vi "X_2.91_main.vi"() -> ()   [LabVIEW 2022 SP3]
panel:
  in  "stop":bool
  in  "Login":bool
  out "Status":string
  out "usr_db":string
  in  "usr":string
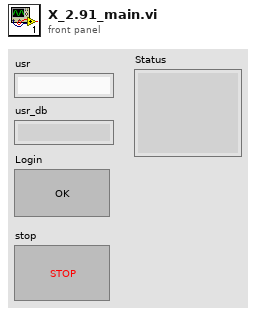
[diagram p1: front panel]
types:
  T1 = enum32{"Invalid", "Standard", "Closed", "Hidden", "Minimized", "Maximized"}
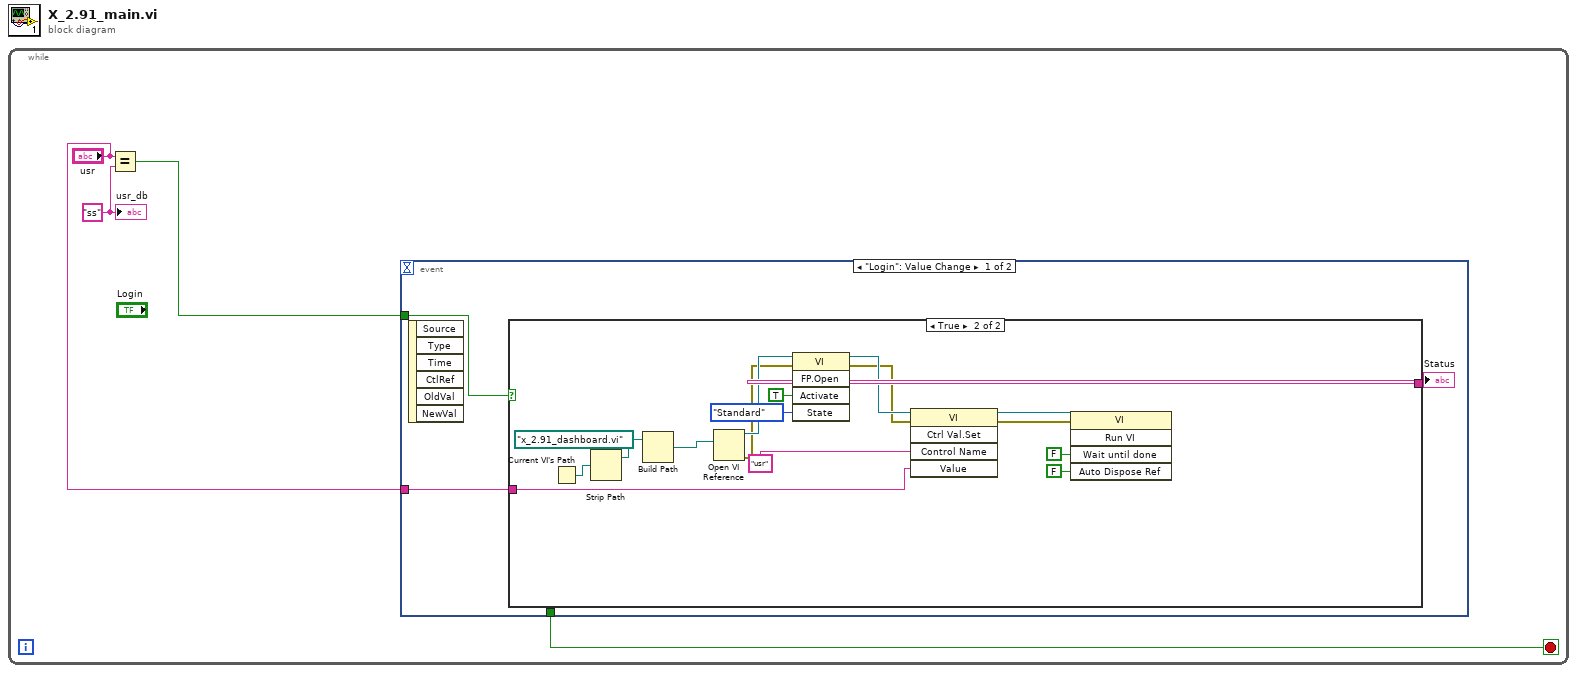
[diagram p0: block diagram]
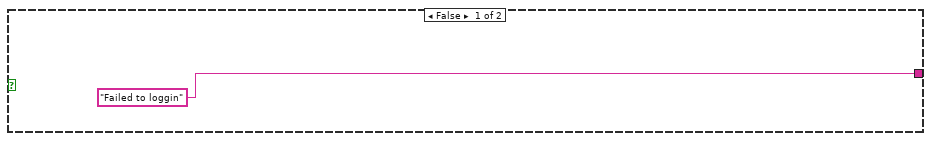
[diagram p2: hidden frame]
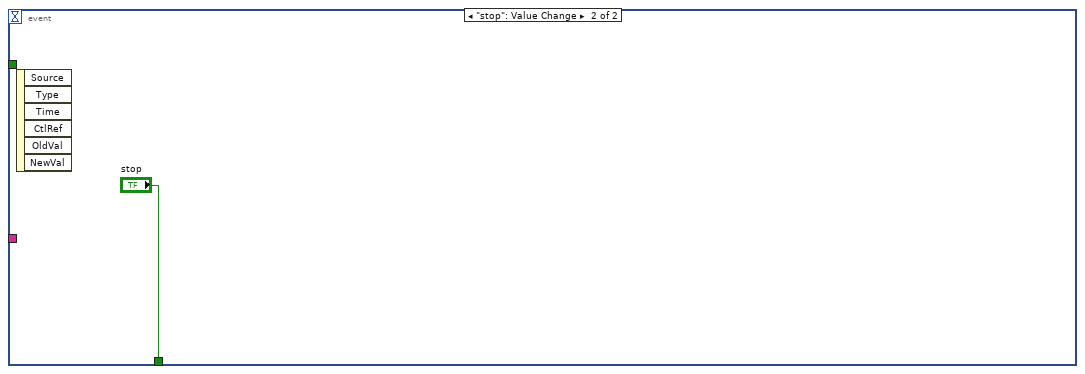
[diagram p3: hidden frame]
diagram:
  n1 = while {
    stop <- w2 stop-if-true
    w4 = "ss"
    n2 = Equal?(x="usr", y=w4) -> (x = y?=w3:bool)
    n3 = event shown="[0] \"Login\": Value Change" {
      selector: _ -> [_ _]
      dyn-events: _ -> [_ _]
      timeout: _ -> [_ _]
      tunnel: w3 -> [w7 _]
      tunnel: [_ "stop"] -> w2
      tunnel: "usr" -> [w5 _]
      event "Login": Value Change {
        n4 = event-data() -> ()  [unwired: 1 in, 6 out]
        n5 = case shown="True" w7 {
          tunnel: ["Failed to loggin" _] -> w6
          tunnel: w5 -> [_ w20]
          frame False {
          }
          frame True {
            n6 = Current VI's Path() -> (path=w24:path)
            n7 = Strip Path(path=w24) -> (stripped path=w23:path)  [unwired: 1 out]
            n8 = Build Path(base path=w23, name or relative path=path "x_2.91_dashboard.vi") -> (appended path=w21:path)
            n9 = Open VI Reference(vi path=w21) -> (vi reference=w14:refnum<vi>, error out=w13:errorcluster)  [unwired: 5 in]
            n10 = invoke class="VI" method="FP.Open"(reference=w14, error in=w13, "Activate"=TRUE ("Activate?"), "State"=T1."Standard") -> (reference out=w12:refnum<vi>, error out=w11:errorcluster)  [unwired: 1 in, 3 out]
            n11 = invoke class="VI" method="Ctrl Val.Set"(reference=w12, error in=w11, "Control Name"="usr", "Value"=w20) -> (reference out=w16:refnum<vi>, error out=w15:errorcluster)  [unwired: 1 in, 3 out]
            n12 = invoke class="VI" method="Run VI"(reference=w16, error in=w15, "Wait until done"=FALSE ("Wait Until Done"), "Auto Dispose Ref"=FALSE ("Auto Dispose Reference")) -> ()  [unwired: 1 in, 5 out]
          }
        }
        "Status" <- w6
      }
      event "stop": Value Change {
        n13 = event-data() -> ()  [unwired: 1 in, 6 out]
      }
    }
    "usr_db" <- w4
  }
